vi "Test Main.vi"() -> ()   [LabVIEW 2018]
uses:
  Classes/STDF File Parser/STDF File Parser.lvclass
  Classes/GRR Core/GRR Core.lvclass
  Classes/Result Display/Result Display.lvclass
  Classes/Process Bar/Process Bar.lvclass
panel:
  out "error out":errorcluster
  in  "STDF Files For Tester#1":path[](array[path])=[path "C:/Users/ziwang/Desktop/0708KGU_V/0708KGU_V/0708KGU_V/KGU_V_1/Hi6M01_A10_V_09May2018_1610.std", path "C:/Users/ziwang/Desktop/0708KGU_V/0708KGU_V/0708KGU_V/KGU_V_2/Hi6M01_A10_V_09May2018_1626.std", path "C:/Users/ziwang/Desktop/0708KGU_V/0708KGU_V/0708KGU_V/KGU_V_3/Hi6M01_A10_V_09May2018_1641.std", path "C:/Users/ziwang/Desktop/0708KGU_V/0708KGU_V/0708KGU_V/KGU_V_4/Hi6M01_A10_V_09May2018_1720.std", path "C:/Users/ziwang/Desktop/0708KGU_V/0708KGU_V/0708KGU_V/KGU_V_5/Hi6M01_A10_V_09May2018_1735.std"]
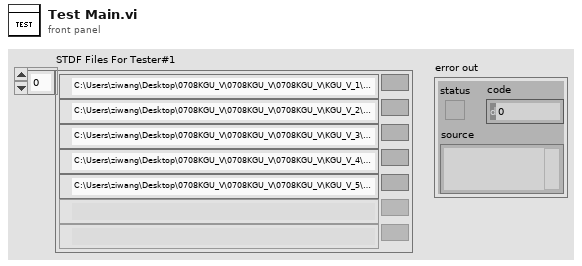
[diagram p1: front panel]
types:
  T1 = typedef "Process Bar.lvclass/Session Handle.ctl" = refnum<data-value>
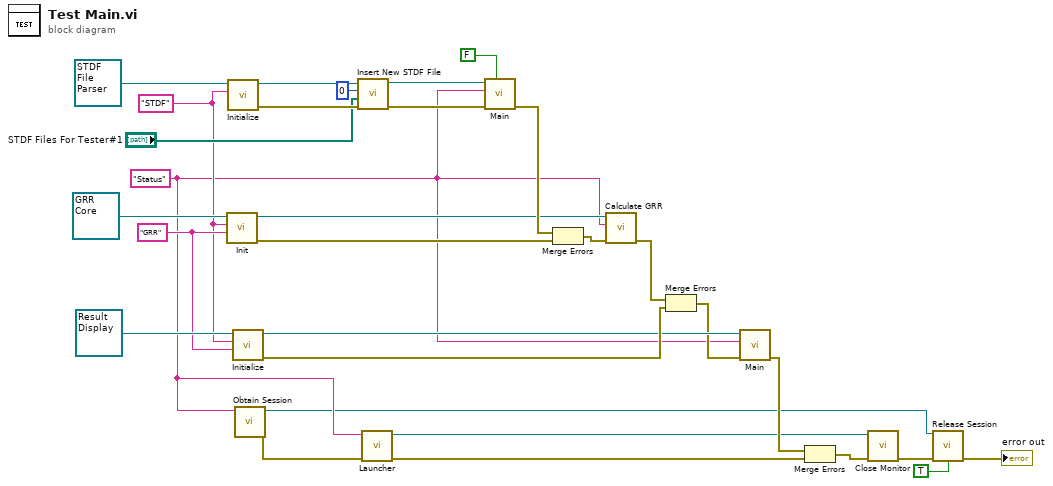
[diagram p0: block diagram]
diagram:
  w16 = "GRR" ("GRR Result Session")
  w9 = "Status" ("Status Monitor")
  w15 = "STDF" ("Parser Name")
  n1 = call "Init.vi"("GRR Result Session"=w16, "STDF Parser"=w15, "GRR Core in"=refnum<class "GRR Core.lvclass"> refnum ("GRR Core.lvclass")) -> ("error out"=w20:errorcluster, "GRR Core out"=w19:refnum<class "GRR Core.lvclass">)  [unwired: 7 in]
  n2 = call "Initialize.vi"("Parser Name"=w15, "STDF File Parser in"=refnum<class "STDF File Parser.lvclass"> refnum ("STDF File Parser.lvclass")) -> ("error out"=w28:errorcluster, "STDF File Parser out"=w29:refnum<class "STDF File Parser.lvclass">)  [unwired: 8 in]
  n3 = call "Initialize.vi"("GRR Data Mgr"=w16, "Test Data Mgr"=w15, "Result Display in"=refnum<class "Result Display.lvclass"> refnum ("Result Display.lvclass")) -> ("error out"=w13:errorcluster, "Result Display out"=w12:refnum<class "Result Display.lvclass">)  [unwired: 7 in]
  n4 = call "Obtain Session.vi"("Session  Name ()"=w9) -> ("error out"=w10:errorcluster, "Session Handle"=w2:T1)  [unwired: 9 in]
  n5 = call "Insert New STDF File.vi"("error in (no error)"=w28, "STDF Files Per Tester"="STDF Files For Tester#1", "Tester #"=u8 0, "STDF File Parser in"=w29) -> ("error out"=w26:errorcluster, "STDF File Parser out"=w27:refnum<class "STDF File Parser.lvclass">)  [unwired: 6 in]
  n6 = call "Launcher.vi"("error in (no error)"=w10, "Session Name"=w9) -> ("error out"=w7:errorcluster, "VI Refnum"=w5:refnum<vi>)  [unwired: 8 in]
  n7 = call "Main.vi"("Check Array Order?"=FALSE, "error in (no error)"=w26, "Status Monitor"=w9, "STDF File Parser in"=w27) -> ("error out"=w21:errorcluster)  [unwired: 6 in, 1 out]
  n8 = Merge Errors(w21, w20) -> (w18:errorcluster)
  n9 = call "Calculate GRR.vi"("error in (no error)"=w18, "Status Monitor"=w9, "GRR Core in"=w19) -> ("error out"=w14:errorcluster)  [unwired: 6 in, 2 out]
  n10 = Merge Errors(w14, w13) -> (w11:errorcluster)
  n11 = call "Main.vi"("error in (no error)"=w11, "Status  Monitor"=w9, "Result Display in"=w12) -> ("error out"=w8:errorcluster)  [unwired: 7 in, 1 out]
  n12 = Merge Errors(w8, w7) -> (w6:errorcluster)
  n13 = call "Close Monitor.vi"("error in (no error)"=w6, "VI Refnum"=w5) -> ("error out"=w4:errorcluster)  [unwired: 9 in]
  n14 = call "Release Session.vi"("Session Handle"=w2, "error in (no error)"=w4, "force destroy? (F)"=TRUE) -> ("error out"=→"error out":errorcluster)  [unwired: 12 in]
